vi "Lookup Node by Name.vi"(8 "error in (no error)":errorcluster, 10 "Name":string, 11 "NodeDiscovery in":refnum<class "DiscoveryService.lvclass">) -> (0 "error out":errorcluster, 2 "Node":T1, 3 "NodeDiscovery out":refnum<class "DiscoveryService.lvclass">)   [LabVIEW 2020, in "Vecto.lvlib" / "DiscoveryService.lvclass"]
uses:
  DiscoveryService.lvclass
  lv-volatus/messages/Discovery/Data.ctl
  lv-volatus/messages/Service/Data.ctl
  lv-volatus/messages/ServiceType/Enumeration.ctl
  DiscoveryService.lvclass/DiscoveryService.ctl
  lv-volatus/messages/ServiceType/ServiceType.lvlib
  lv-volatus/messages/Service/Service.lvlib
  lv-volatus/messages/Discovery/Discovery.lvlib
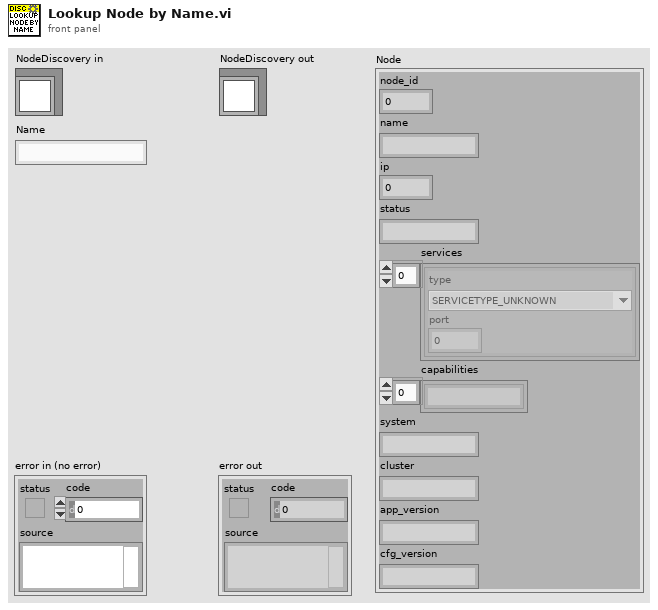
[diagram p1: front panel]
types:
  T1 = typedef "Discovery.lvlib/Data.ctl" = cluster{"node_id":u32, "name":string, "ip":u32, "status":string, "services":T2[], "capabilities":string[], "system":string, "cluster":string, "app_version":string, "cfg_version":string}
  T2 = typedef "Service.lvlib/Data.ctl" = cluster{"type":T3, "port":i32}
  T3 = typedef "ServiceType.lvlib/Enumeration.ctl" = enum16{"SERVICETYPE_UNKNOWN", "SERVICETYPE_TCPSERVER", "SERVICETYPE_HTTPSERVER"}
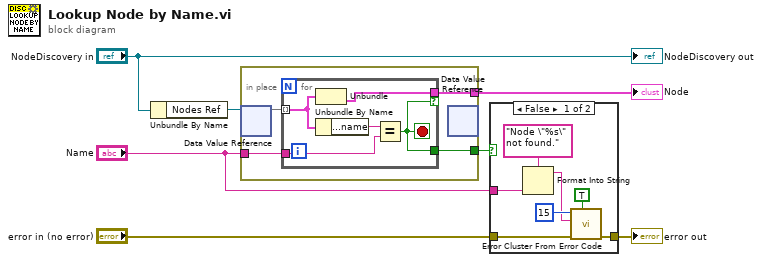
[diagram p0: block diagram]
diagram:
  n1 = Unbundle By Name("NodeDiscovery in") -> ("Nodes Ref"=w6:refnum<data-value>)
  n2 = in-place {
    in-place-border: "Name" -> [w10]
    in-place-border: [w9] -> w4
    in-place-border: [w8] -> w5
    n3 = in-place-dvr #1(w6) -> (w11:map{u32, T1})  [unwired: 1 out]
    n4 = for {
      tunnel: w11 -> [w16] mode=indexing
      tunnel: w10 -> [w14]
      tunnel: [w12] -> w9 if=w13
      tunnel: [w13] -> w8
      stop <- w13 stop-if-true
      n5 = Unbundle(w16) -> ("Discovery"=w12:T1)  [unwired: 1 out]
      n6 = Unbundle By Name(w16) -> ("Discovery.name"=w15:string)
      n7 = Equal?(x=w15, y=w14) -> (x = y?=w13:bool)
    }
    n8 = in-place-dvr #1() -> ()  [unwired: 1 in, 2 out]
  }
  "Node" <- w4
  n9 = case shown="False" w5 {
    tunnel: "Name" -> [w21 _]
    tunnel: "error in (no error)" -> [w18 w24]
    tunnel: [w17 w24] -> w1
    frame False {
      n10 = Format Into String(format string="Node \"%s\" not found.", w21) -> (resulting string=w19:string)  [unwired: 2 in, 1 out]
      n11 = call <vilib>:"Error Cluster From Error Code.vi"("show call chain? (False)"=TRUE, "error in (no error)"=w18, "error message (\"\")"=w19, "error code (0)"=15) -> ("error out"=w17:errorcluster)  [unwired: 5 in]
    }
    frame True {
    }
  }
  "error out" <- w1
  "NodeDiscovery out" <- "NodeDiscovery in"
